vi "99%BW.vi"() -> ()   [LabVIEW 2016]
panel:
  in  "VISA resource name":refnum<visa-resource-name>
  in  "Occupied Bandwidth Centre frequency(MHz)":dbl=99.0 format="%#.6g"
  in  "X dB (-26 dB)":dbl=-26.0 format="%#.6g"
  in  "Occupied Bandwidth Span (MHz)":dbl=3000000.0 format="%#.6g"
  in  "Max Hold (OFF)":bool
  in  "Occupied Bandwidth Percent Power (99%)":dbl=99.0 format="%#.6g"
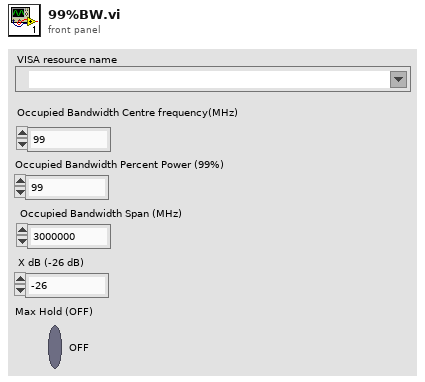
[diagram p1: front panel]
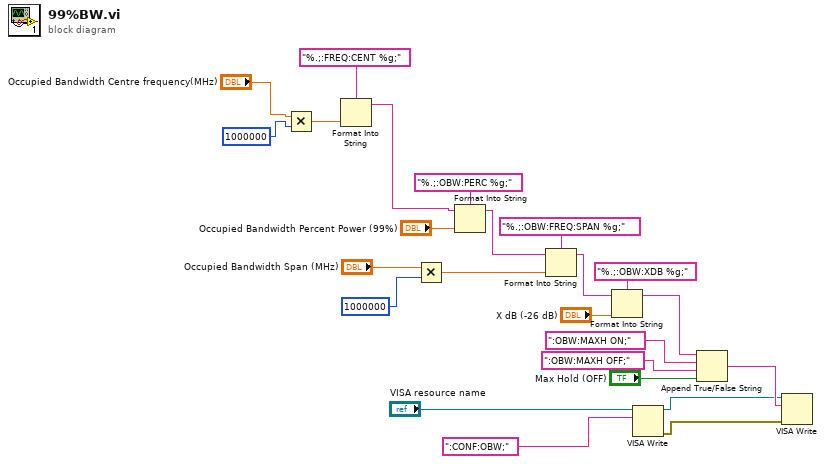
[diagram p0: block diagram]
diagram:
  n1 = Multiply(x="Occupied Bandwidth Centre frequency(MHz)", y=1000000) -> (x*y=w11:dbl)
  n2 = Format Into String(format string="%.;:FREQ:CENT %g;", w11) -> (resulting string=w7:string)  [unwired: 2 in, 1 out]
  n3 = Multiply(x="Occupied Bandwidth Span (MHz)", y=1000000) -> (x*y=w8:dbl)
  n4 = Format Into String(format string="%.;:OBW:PERC %g;", initial string=w7, "Occupied Bandwidth Percent Power (99%)") -> (resulting string=w21:string)  [unwired: 1 in, 1 out]
  n5 = Format Into String(format string="%.;:OBW:FREQ:SPAN %g;", initial string=w21, w8) -> (resulting string=w18:string)  [unwired: 1 in, 1 out]
  n6 = Format Into String(format string="%.;:OBW:XDB %g;", initial string=w18, "X dB (-26 dB)") -> (resulting string=w14:string)  [unwired: 1 in, 1 out]
  n7 = VISA Write(VISA resource name="VISA resource name", write buffer=":CONF:OBW;" ("initial string")) -> (VISA resource name out=w2:refnum<visa-resource-name>, error out=w1:errorcluster)  [unwired: 1 in, 1 out]
  n8 = Append True/False String(1:"Max Hold (OFF)", 2:":OBW:MAXH OFF;", 3:":OBW:MAXH ON;", 4:w14) -> (0:w5:string)
  n9 = VISA Write(VISA resource name=w2, write buffer=w5, error in (no error)=w1) -> ()  [unwired: 3 out]
